vi "AdmittanceFilter.vi"(8 "error in (no error)":errorcluster, 9 "Fy":dbl, 10 "Fx":dbl, 11 "AdmittanceCoeffs":T1={"C"=1.0, "k"=1.0}) -> (0 "error out":errorcluster, 1 "Delta y":dbl, 2 "Delta x":dbl)   [LabVIEW 2017, in "admittanceControllerLibrary.lvlib"]
uses:
  admittanceControllerLibrary.lvlib
  Controls/AdmittanceGains.ctl
  <vilib>/imath/engines/lvmath2/RunTimeEngine/NodeEndStatement/NIMS_NodeEndStatement_Output.vi
  <instcachedir>/0/NIMS_NodeEndStatement_Output_53EC0D466D134D7ABD903AC30B43404B.lvgen/NIMS_NodeEndStatement_Output_53EC0D466D134D7ABD903AC30B43404B_001.vi
  <vilib>/imath/engines/lvmath2/RunTimeEngine/ErrorHandling/NIMS_Finalize Error.vi
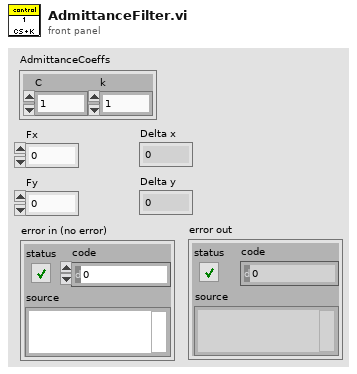
[diagram p1: front panel]
types:
  T1 = typedef "admittanceControllerLibrary.lvlib/AdmittanceGains.ctl" = cluster{"C":dbl, "k":dbl}
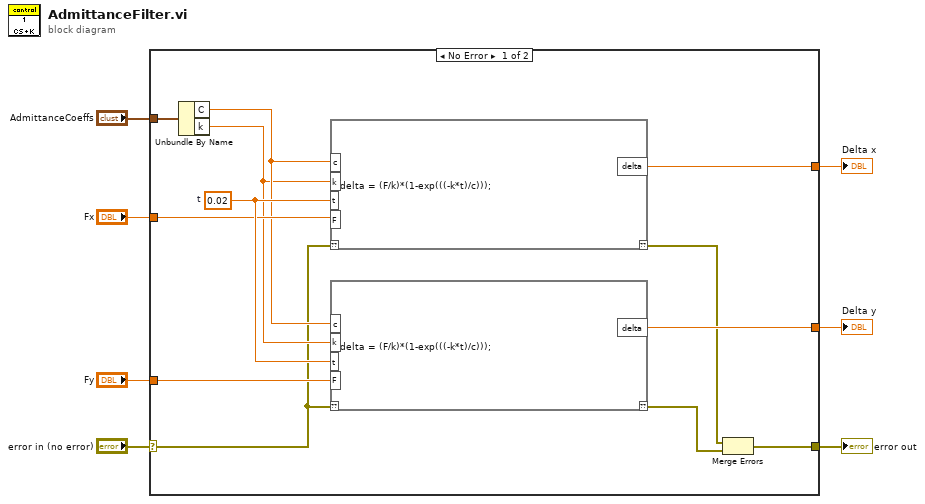
[diagram p0: block diagram]
diagram:
  n1 = case shown="No Error" "error in (no error)" {
    selector: "error in (no error)" -> [w11 w86]
    tunnel: [w19 _] -> w7
    tunnel: "Fx" -> [w17 _]
    tunnel: "Fy" -> [w16 _]
    tunnel: [w15 _] -> w4
    tunnel: "AdmittanceCoeffs" -> [w14 _]
    tunnel: [w8 w86] -> w1
    frame No Error {
      w18 = 0.02  # t
      n2 = Unbundle By Name(w14) -> ("C"=w13:dbl, "k"=w12:dbl)
      n3 = mathscript code="delta = (F/k)*(1-exp(((-k*t)/c)));"("??"=w11, "F"=w17, "c"=w13, "k"=w12, "t"=w18) -> ("??"=w10:errorcluster, "delta"=w19:dbl)
      n4 = mathscript code="delta = (F/k)*(1-exp(((-k*t)/c)));"("??"=w11, "F"=w16, "c"=w13, "k"=w12, "t"=w18) -> ("??"=w9:errorcluster, "delta"=w15:dbl)
      n5 = Merge Errors(w10, w9) -> (w8:errorcluster)
    }
    frame Error {
    }
  }
  "Delta x" <- w7
  "Delta y" <- w4
  "error out" <- w1
